vi "FlipFlop.vi"(1 "input":bool, 2 "clock":bool) -> (0 "output":bool)   [LabVIEW 2012]
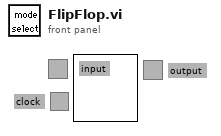
[diagram p1: front panel]
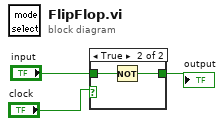
[diagram p0: block diagram]
diagram:
  n1 = case shown="True" "clock" {
    tunnel: "input" -> [w4 w6]
    tunnel: [w4 w5] -> w1
    frame False {
    }
    frame True {
      n2 = Not(x=w6) -> (.not. x?=w5:bool)
    }
  }
  "output" <- w1
